vi "Splitsen.vi"() -> ()   [LabVIEW 2024]
panel:
  out "Afstand":dbl
  in  "input string":string
  out "Humdity":dbl
  out "Temperatuur":dbl
  out "Hic":dbl
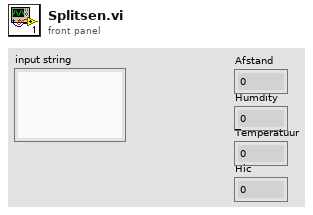
[diagram p1: front panel]
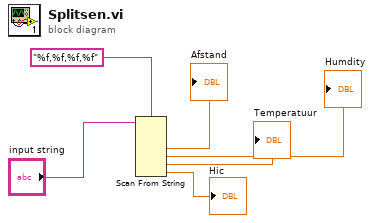
[diagram p0: block diagram]
diagram:
  n1 = Scan From String(format string="%f,%f,%f,%f" ("input string"), input string="input string") -> (output 1=→"Afstand":dbl, output 2=→"Humdity":dbl, output 3=→"Temperatuur":dbl, output 4=→"Hic":dbl)  [unwired: 6 in, 3 out]
